vi "Configure SRL Connector Port.vi"(6 "Capacity (0 F)":dbl, 7 "Connector Length (0 m)":dbl, 8 "error in (no error)":errorcluster, 9 "Port (1)":i32=1, 10 "Channel (1)":i32=1, 11 "VISA resource name":refnum<visa-resource-name>) -> (0 "error out":errorcluster, 3 "VISA resource name out":refnum<visa-resource-name>)   [LabVIEW 2022 SP3, in "Agilent ENA Series.lvlib"]
doc: "Configures SRL measurement port.\n\n<B>Note:</B>This VI is only vaild on E5061B."
uses:
  <instrlib>/Agilent ENA Series/Agilent ENA Series.lvlib
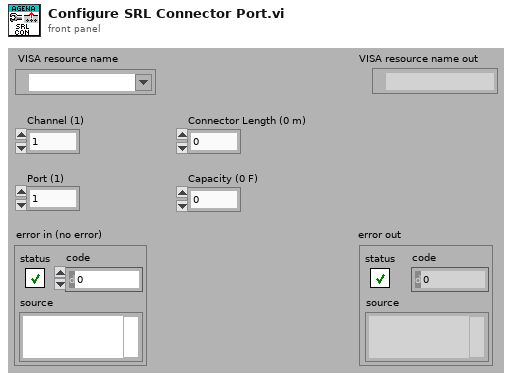
[diagram p1: front panel]
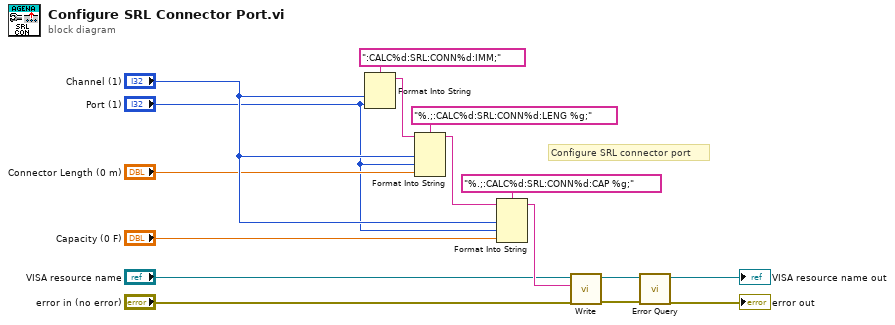
[diagram p0: block diagram]
diagram:
  # "Configure SRL connector port"
  n1 = Format Into String(format string=":CALC%d:SRL:CONN%d:IMM;", "Channel (1)", "Port (1)") -> (resulting string=w6:string)  [unwired: 2 in, 1 out]
  n2 = Format Into String(format string="%.;:CALC%d:SRL:CONN%d:LENG %g;", initial string=w6, "Channel (1)", "Port (1)", "Connector Length (0 m)") -> (resulting string=w12:string)  [unwired: 1 in, 1 out]
  n3 = Format Into String(format string="%.;:CALC%d:SRL:CONN%d:CAP %g;", initial string=w12, "Channel (1)", "Port (1)", "Capacity (0 F)") -> (resulting string=w5:string)  [unwired: 1 in, 1 out]
  n4 = call <instrlib>:"Write.vi"("error in (no error)"="error in (no error)", "String ()"=w5, "VISA resource name"="VISA resource name") -> ("error out"=w1:errorcluster, "VISA resource name out"=w2:refnum<visa-resource-name>)  [unwired: 6 in, 1 out]
  n5 = call <instrlib>:"Error Query.vi"("error in (no error)"=w1, "VISA resource name"=w2) -> ("error out"=→"error out":errorcluster, "VISA resource name out"=→"VISA resource name out":refnum<visa-resource-name>)  [unwired: 8 out]
